vi "lsl pull sample l.vi"(0 "in":cluster{}, 1 "ec":i32, 5 "buffer":i32, 7 "buffer_elements":i32, 9 "timeout":dbl, 11 "error in (no error)":errorcluster) -> (3 "ec out":i32, 4 "in out":cluster{}, 6 "buffer out":i32, 8 "function return":dbl, 15 "error out":errorcluster)   [LabVIEW 2018, in "liblsl-LabVIEW.lvlib"]
doc: "extern LIBLSL_C_API double lsl_pull_sample_l(lsl_inlet in, long *buffer, int buffer_elements, double timeout, int *ec);"
uses:
  <userlib>/liblsl-LabVIEW/liblsl-LabVIEW.lvlib
  <userlib>/liblsl-LabVIEW/liblsl64.dll
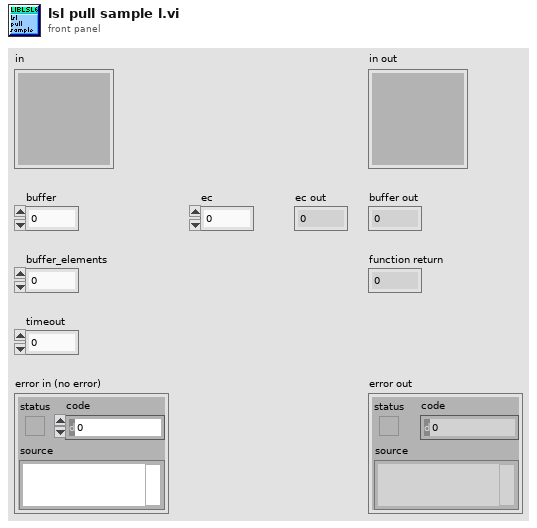
[diagram p1: front panel]
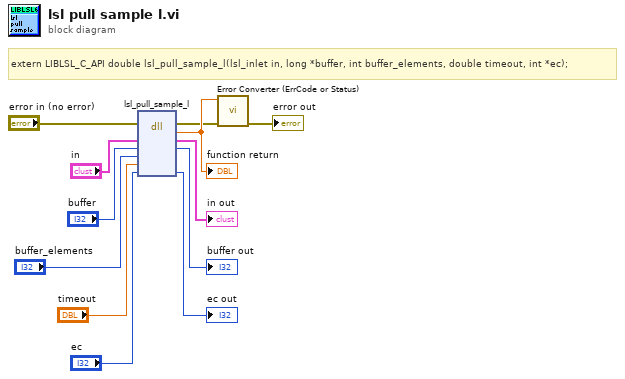
[diagram p0: block diagram]
diagram:
  # "extern LIBLSL_C_API double lsl_pull_sample_l(lsl_inlet in, long *buffer, int buffer_elements, double timeout, int *ec);"
  n1 = dll-call lib="C:/Program Files/National Instruments/LabVIEW 2018/user.lib/liblsl-LabVIEW/liblsl64.*" fn="lsl_pull_sample_l"(error in="error in (no error)", "in"="in", "buffer"="buffer", "buffer_elements"="buffer_elements", "timeout"="timeout", "ec"="ec") -> (error out=w2:errorcluster, w12:dbl, "in"=→"in out":cluster{}, "buffer"=→"buffer out":i32, "ec"=→"ec out":i32)  [unwired: 4 in, 1 out]
  "function return" <- w12
  n2 = call <userlib>:"Error Converter (ErrCode or Status).vi"("error in (no error)"=w2, "error code"=w12) -> ("error out"=→"error out":errorcluster)  [unwired: 9 in]
